vi "NI32LV223f0ASD3_Untitled 2.vi"() -> ()   [LabVIEW 2022 SP3]
panel:
  in  "Numeric":dbl
  out "XY Graph":cluster{"X":dbl, "Y":dbl}[](graph)
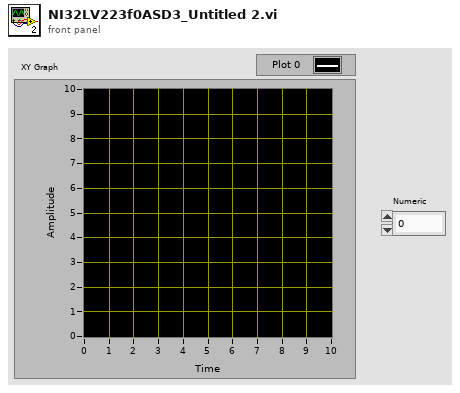
[diagram p1: front panel]
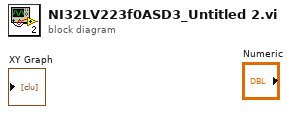
[diagram p0: block diagram]
diagram:
